vi "ep_Time Calculation.vi"(5 "definite reset? (F)":bool, 6 "reset delay [s]":dbl, 7 "time dial":dbl=1.0, 8 "error in (no error)":errorcluster, 9 "operate time compensation":cluster{"G/Gs":dbl, "compensation [s]":dbl}[](array[cluster]), 10 "curve parameters":T1={"operate time parameters"={"A [s]"=1.0, "B [s]"=1.0, "alpha"=1.0, "K2 [s]"=1.0, "K1 [s]"=1.0, "K3 [s]"=1.0}, "reset time parameters"={"tr [s]"=1.0, "alpha"=1.0}}, 11 "GD":u16=25) -> (0 "error out":errorcluster, 1 "memory size":u16, 3 "memory initial values":fxp<+,50,50>[](array[numeric]), 4 "curve data":cluster{"G/Gs":dbl[], "times":dbl[]})   [LabVIEW 2012, in "NI_EP_Protection.lvlib"]
uses:
  <vilib>/addons/Electrical Power/Protection/NI_EP_Protection.lvlib
  <vilib>/addons/Electrical Power/Protection/Inverse Time Delay/subVIs/ep_Curve Parameters.ctl
  <vilib>/addons/Electrical Power/Protection/Inverse Time Delay/subVIs/ep_Operate Time.ctl
  <vilib>/addons/Electrical Power/Protection/Inverse Time Delay/subVIs/ep_Reset Time.ctl
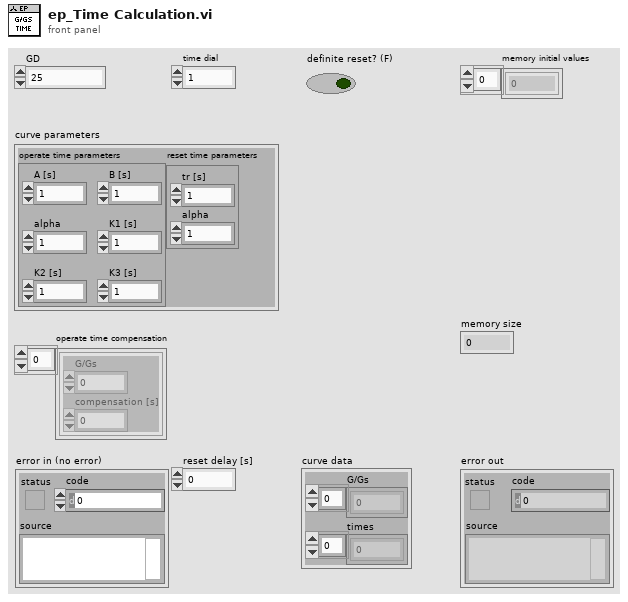
[diagram p1: front panel]
types:
  T1 = typedef "NI_EP_Protection.lvlib/ep_Curve Parameters.ctl" = cluster{"operate time parameters":T2, "reset time parameters":T3}
  T2 = typedef "NI_EP_Protection.lvlib/ep_Operate Time.ctl" = cluster{"A [s]":dbl, "B [s]":dbl, "alpha":dbl, "K2 [s]":dbl, "K1 [s]":dbl, "K3 [s]":dbl}
  T3 = typedef "NI_EP_Protection.lvlib/ep_Reset Time.ctl" = cluster{"tr [s]":dbl, "alpha":dbl}
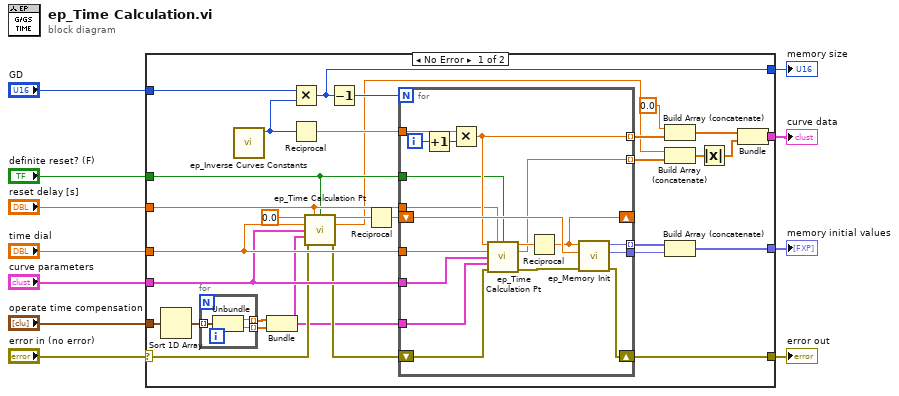
[diagram p0: block diagram]
diagram:
  n1 = case shown="No Error" "error in (no error)" {
    selector: "error in (no error)" -> [w36 w64]
    tunnel: "curve parameters" -> [w37 _]
    tunnel: "time dial" -> [w38 _]
    tunnel: "GD" -> [w42 _]
    tunnel: [w23 _] -> w5
    tunnel: [w41 _] -> w9
    tunnel: [w33 w64] -> w7
    tunnel: [w25 _] -> w6
    tunnel: "reset delay [s]" -> [w19 _]
    tunnel: "definite reset? (F)" -> [w18 _]
    tunnel: "operate time compensation" -> [w17 _]
    frame No Error {
      n2 = Sort 1D Array(array=w17) -> (sorted array=w16:cluster{"G/Gs":dbl, "compensation [s]":dbl}[])
      n3 = for {
        tunnel: w16 -> [w45] mode=indexing
        tunnel: [w44] -> w15 mode=indexing
        tunnel: [w43] -> w14 mode=indexing
        n4 = Unbundle(w45) -> ("G/Gs"=w44:dbl, "compensation [s]"=w43:dbl)
      }
      n5 = call <vilib>:"ep_Inverse Curves Constants.vi"() -> ("number of sections in each G/Gs step"=w39:u16)  [unwired: 6 in, 5 out]
      n6 = Bundle(w15, w14) -> (w13:cluster{dbl[], dbl[]})  [unwired: 1 in]
      n7 = Multiply(x=w42, y=w39) -> (x*y=w41:u16)
      n8 = Reciprocal(x=w39) -> (1/x=w40:dbl)
      n9 = call <vilib>:"ep_Time Calculation Pt.vi"("multiples of pickup"=0.0, "reset delay [s]"=w19, "definite reset? (F)"=w18, "time dial"=w38, "curve parameters"=w37, "operate time compensation"=w13, "error in (no error)"=w36) -> ("compensated time"=w28:dbl, "original time"=w12:dbl, "error out"=w35:errorcluster)  [unwired: 6 in]
      n10 = Decrement(x=w41) -> (x-1=w34:u16)
      n11 = Reciprocal(x=w28) -> (1/x=w20:dbl)
      n12 = for {
        N: w34 -> [_]
        tunnel: w37 -> [w59]
        tunnel: w38 -> [w60]
        tunnel: [w56] -> w24 mode=indexing
        tunnel: w40 -> [w63]
        shift-right: [w55] -> w33
        shift-left: w35 -> [w58]
        shift-right: [w50] -> _
        shift-left: w20 -> [w54]
        tunnel: [w46] -> w31 mode=indexing
        tunnel: [w52] -> w30 mode=indexing
        tunnel: [w51] -> w22
        tunnel: w19 -> [w49]
        tunnel: w18 -> [w48]
        tunnel: w13 -> [w47]
        i -> [w62]
        n13 = Increment(x=w62) -> (x+1=w61:i32)
        n14 = Multiply(x=w63, y=w61) -> (x*y=w52:dbl)
        n15 = call <vilib>:"ep_Time Calculation Pt.vi"("multiples of pickup"=w52, "reset delay [s]"=w49, "definite reset? (F)"=w48, "time dial"=w60, "curve parameters"=w59, "operate time compensation"=w47, "error in (no error)"=w58) -> ("compensated time"=w53:dbl, "original time"=w46:dbl, "error out"=w57:errorcluster)  [unwired: 6 in]
        n16 = Reciprocal(x=w53) -> (1/x=w50:dbl)
        n17 = call <vilib>:"ep_Memory Init.vi"("error in (no error)"=w57, "1/previous time"=w54, "1/time"=w50) -> ("error out"=w55:errorcluster, "last memory initial value"=w51:fxp<+,50,50>, "memory initial value"=w56:fxp<+,50,50>)  [unwired: 6 in]
      }
      n18 = Build Array (concatenate)(0.0 ("multiples of pickup"), w30) -> (w27:dbl[])
      n19 = Build Array (concatenate)(w12, w31) -> (w26:dbl[])
      n20 = Build Array (concatenate)(w24, w22) -> (w23:fxp<+,50,50>[])
      n21 = Absolute Value(x=w26) -> (abs(x)=w21:dbl[])
      n22 = Bundle(w27, w21) -> (w25:cluster{dbl[], dbl[]})  [unwired: 1 in]
    }
    frame Error {
    }
  }
  "memory size" <- w9
  "error out" <- w7
  "curve data" <- w6
  "memory initial values" <- w5
